vi "ASDA-A2_Session.vi"(6 "Get/Set (T=Set)":bool, 8 "error in":errorcluster, 10 "Session In":refnum<class "Modbus Master.lvclass">, 11 "Buffer Data In":T1) -> (0 "error out":errorcluster, 2 "Session Out":refnum<class "Modbus Master.lvclass">, 3 "Buffer Data Out":T1)   [LabVIEW 2016]
uses:
  Data Def/ASDA-A2_Buffer Data.ctl
  <vilib>/Modbus/master/Modbus Master.lvclass
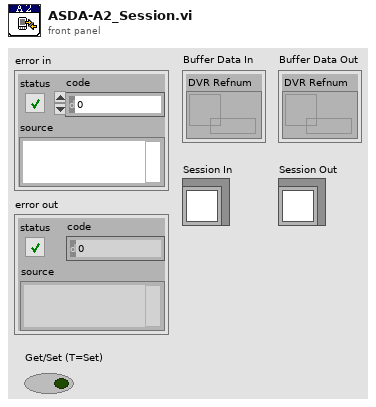
[diagram p1: front panel]
types:
  T1 = typedef "ASDA-A2_Buffer Data.ctl" = cluster{"DVR Refnum":refnum<data-value>}
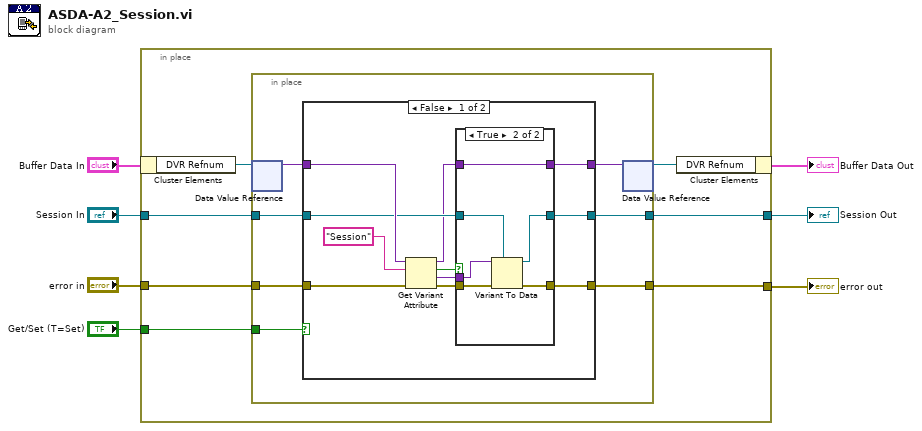
[diagram p0: block diagram]
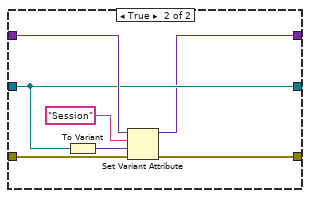
[diagram p3: hidden frame]
diagram:
  n1 = in-place {
    in-place-border: "Get/Set (T=Set)" -> [w12]
    in-place-border: "error in" -> [w11]
    in-place-border: "Session In" -> [w10]
    in-place-border: [w9] -> w1
    in-place-border: [w8] -> w2
    n2 = in-place-cluster #1("Buffer Data In") -> ("DVR Refnum"=w14:refnum<data-value>)
    n3 = in-place {
      in-place-border: w12 -> [w21]
      in-place-border: w11 -> [w19]
      in-place-border: w10 -> [w18]
      in-place-border: [w17] -> w9
      in-place-border: [w15] -> w8
      n4 = in-place-dvr #2(w14) -> (w20:variant)  [unwired: 1 out]
      n5 = case shown="False" w21 {
        tunnel: w20 -> [w32 w47]
        tunnel: w19 -> [w31 w48]
        tunnel: w18 -> [w27 w44]
        tunnel: [w26 w44] -> w17
        tunnel: [w23 w42] -> w16
        tunnel: [w22 w43] -> w15
        frame False {
          n6 = Get Variant Attribute(Variant=w32, name="Session", error in=w31) -> (duplicate Variant=w25:variant, found=w29:bool, value=w24:variant, error out=w28:errorcluster)  [unwired: 1 in]
          n7 = case shown="True" w29 {
            tunnel: w28 -> [w33 w41]
            tunnel: w27 -> [w35 w40]
            tunnel: [w35 w39] -> w26
            tunnel: w25 -> [w34 w37]
            tunnel: w24 -> [_ w38]
            tunnel: [w34 w37] -> w23
            tunnel: [w33 w36] -> w22
            frame False {
            }
            frame True {
              n8 = Variant To Data(error in=w41, type=w40, Variant=w38) -> (data=w39:refnum<class "Modbus Master.lvclass">, error out=w36:errorcluster)
            }
          }
        }
        frame True {
          n9 = To Variant(anything=w44) -> (Variant=w45:variant)
          n10 = Set Variant Attribute(Variant=w47, name="Session", value=w45, error in=w48) -> (Variant out=w42:variant, error out=w43:errorcluster)  [unwired: 1 out]
        }
      }
      n11 = in-place-dvr #2(w16) -> (w13:refnum<data-value>)  [unwired: 1 out]
    }
    n12 = in-place-cluster #1("DVR Refnum"=w13) -> (→"Buffer Data Out":T1)
  }
  "error out" <- w2
  "Session Out" <- w1
